vi "Publish Rack Status.vi"(8 "Error In":errorcluster, 11 "KIT-QVA in":refnum<class "KIT-QVA.lvclass">) -> (0 "Error Out":errorcluster, 3 "KIT-QVA out":refnum<class "KIT-QVA.lvclass">)   [LabVIEW 2014, in "KIT-QVA.lvlib" / "KIT-QVA.lvclass"]
doc: "Publish rack status."
uses:
  KIT-QVA.lvclass
  KIT-QVA.lvclass/KIT-QVA.ctl
  RackStatus-PVEnum.ctl
  CSPP_Core/Classes/CS++ProcessVariables/PVConnection/PVConnection.lvclass/PVConnection.ctl
  CSPP_Core/Classes/CS++ProcessVariables/ProcessVariable/PV.lvclass/PV.ctl
  CSPP_Core/Classes/CS++ProcessVariables/ProcessVariable/Write Data.vi
  CSPP_Core/Classes/CS++ProcessVariables/ProcessVariable/Write Timestamp.vi
  CSPP_Core/Classes/CS++ProcessVariables/ProcessVariable/Write Quality.vi
  CSPP_Core/Classes/CS++ProcessVariables/ProcessVariable/Write status.vi
  CSPP_Core/Classes/CS++ProcessVariables/ProcessVariable/Write Error.vi
  CSPP_Core/Classes/CS++ProcessVariables/ProcessVariable/PV.lvclass
  CSPP_Core/Classes/CS++ProcessVariables/PVConnection/PVConnection.lvclass
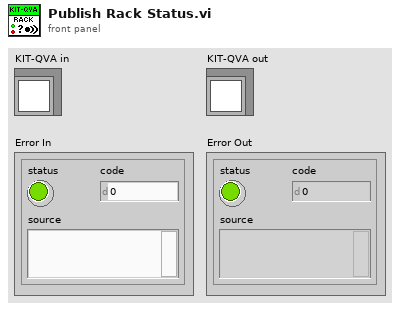
[diagram p1: front panel]
types:
  T1 = cluster{"System Test":bool, "Test Mode":bool, "Fault":bool, "Quench":bool, "U/T Fault":bool, "Bus Error":bool, "System Fault":bool, "Control Mode":bool}
  T2 = typedef "KIT-QVA.lvlib/KIT-QVA.lvclass/RackStatus-PVEnum.ctl" = enum16{"RS-SystemTest", "RS-TestMode", "RS-Fault", "RS-Quench", "RS-UTFault", "RS-BusError", "RS-SystemFault", "RS-ControlMode", "RS-AveragedT"}
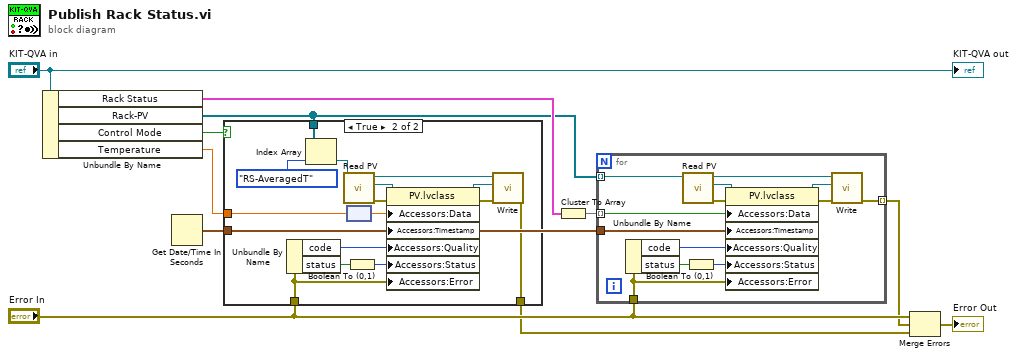
[diagram p0: block diagram]
diagram:
  n1 = Unbundle By Name("KIT-QVA in") -> ("Rack Status"=w9:T1, "Rack-PV"=w7:refnum<class "PVConnection.lvclass">[], "Control Mode"=w1:bool, "Temperature"=w10:dbl[unit])
  n2 = Get Date/Time In Seconds() -> (seconds since 1Jan1904=w6:timestamp)
  n3 = case shown="True" w1 {
    tunnel: w10 -> [_ w21]
    tunnel: w7 -> [_ w17]
    tunnel: w6 -> [_ w16]
    tunnel: "Error In" -> [w12 w15]
    tunnel: [w12 w14] -> w2
    frame False {
    }
    frame True {
      n4 = Unbundle By Name(w15) -> ("code"=w23:i32, "status"=w24:bool)
      n5 = Index Array(array=w17, index=RackStatus-PVEnum."RS-AveragedT" ("Rack-PVEnum")) -> (element=w27:refnum<class "PVConnection.lvclass">)
      n6 = call "Read PV.vi"("PVConnection in"=w27) -> ("error out"=w25:errorcluster, "PV"=w26:refnum<class "PV.lvclass">, "PVConnection out"=w19:refnum<class "PVConnection.lvclass">)  [unwired: 8 in]
      n7 = node(w21) -> (w13:dbl)
      n8 = Boolean To (0,1)(Boolean=w24) -> (0, 1=w22:i16)
      n9 = property class="PV.lvclass"(reference=w26, error in=w25, "Accessors:Data"=w13, "Accessors:Timestamp"=w16, "Accessors:Quality"=w23, "Accessors:Status"=w22, "Accessors:Error"=w15) -> (reference out=w20:refnum<class "PV.lvclass">, error out=w18:errorcluster)
      n10 = call "Write.vi"("error in (no error)"=w18, "PV"=w20, "PVConnection in"=w19) -> ("error out"=w14:errorcluster)  [unwired: 7 in, 1 out]
    }
  }
  n11 = Cluster To Array(cluster=w9) -> (array=w8:bool[])
  n12 = for {
    tunnel: w8 -> [w33] mode=indexing
    tunnel: w7 -> [w32] mode=indexing
    tunnel: w6 -> [w31]
    tunnel: "Error In" -> [w30]
    tunnel: [w29] -> w3 mode=indexing
    n13 = Unbundle By Name(w30) -> ("code"=w37:i32, "status"=w36:bool)
    n14 = call "Read PV.vi"("PVConnection in"=w32) -> ("error out"=w35:errorcluster, "PV"=w34:refnum<class "PV.lvclass">, "PVConnection out"=w40:refnum<class "PVConnection.lvclass">)  [unwired: 8 in]
    n15 = Boolean To (0,1)(Boolean=w36) -> (0, 1=w38:i16)
    n16 = property class="PV.lvclass"(reference=w34, error in=w35, "Accessors:Data"=w33, "Accessors:Timestamp"=w31, "Accessors:Quality"=w37, "Accessors:Status"=w38, "Accessors:Error"=w30) -> (reference out=w39:refnum<class "PV.lvclass">, error out=w41:errorcluster)
    n17 = call "Write.vi"("error in (no error)"=w41, "PV"=w39, "PVConnection in"=w40) -> ("error out"=w29:errorcluster)  [unwired: 7 in, 1 out]
  }
  n18 = Merge Errors("Error In", w3, w2) -> (→"Error Out":errorcluster)
  "KIT-QVA out" <- "KIT-QVA in"
